vi "Spreadsheet_storage.vi"(9 "Waveform Parameters":T1, 10 "Digitizing Parameters":T2) -> (1 "Waveform Output":cluster{"t":dbl[], "x":dbl[]})   [LabVIEW 2015]
uses:
  <vilib>/Utility/file.llb/Write Delimited Spreadsheet (DBL).vi
panel:
  out "XY Graph":cluster{"t":dbl[], "x":dbl[]}(graph)
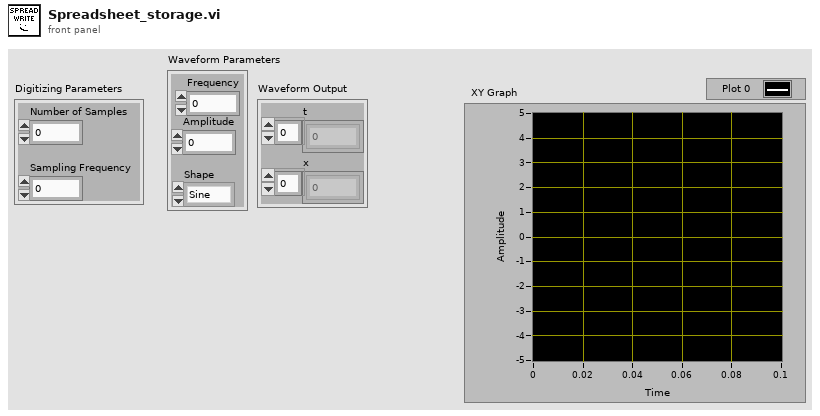
[diagram p1: front panel]
types:
  T1 = cluster{"Frequency":dbl, "Amplitude":dbl, "Shape":enum16{"Sine", "Cosine", "DC Level", "Square", "User-Defined"}}
  T2 = cluster{"Number of Samples":dbl, "Sampling Frequency":dbl}
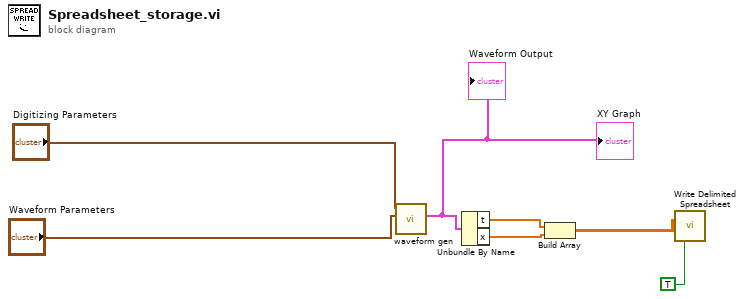
[diagram p0: block diagram]
diagram:
  n1 = call "waveform gen.vi"("Waveform Parameters"="Waveform Parameters", "Digitizing Parameters"="Digitizing Parameters") -> ("Waveform Output"=w1:cluster{"t":dbl[], "x":dbl[]})  [unwired: 9 in]
  "XY Graph" <- w1
  "Waveform Output" <- w1
  n2 = Unbundle By Name(w1) -> ("t"=w5:dbl[], "x"=w4:dbl[])
  n3 = Build Array(w5, w4) -> (w3:dbl[][])
  n4 = call-poly <vilib>:"Write Delimited Spreadsheet.vi"("2D data"=w3, "transpose? (F)"=TRUE) -> ()  [unwired: 12 in, 2 out]
